vi "MMI_BCM_2A1_Action.vi"(8 "error in":errorcluster caption="错误输入", 9 "Input2":T1, 10 "Input1":T2, 11 "BCM":T3 {"语音命令天窗开关" items=["默认", "停止"]; "天窗开度" scale=0.0..100.0; "右后侧车窗开度" scale=0.0..100.0; "左后侧车窗开度" scale=0.0..100.0; "副驾驶侧车窗开度" scale=0.0..100.0; "伴我回家时间" items=["无", "30s", "60s", "90s"]; "门解锁设置应答" items=["无应答", "应答驾驶门解锁", "应答所有门解锁"]; "天窗翘起控制" items=["无", "倾斜翘起", "倾斜关闭"]; "车窗防夹报警" items=["无", "禁止", "启用"]; "日间行车灯" items=["无", "禁止", "启用"]; "智能弯道灯" items=["无", "禁止", "启用"]; "后视镜自动折叠" items=["无", "禁止", "启用"]; "下雨关窗模式" items=["无", "关", "开"]; "设防提示类型" items=["无", "亮灯并鸣笛", "亮灯", "鸣笛"]; "驾驶侧车窗开度" scale=0.0..100.0}) -> (0 "error out":errorcluster caption="错误输出")   [LabVIEW 2013]
uses:
  MMI_BCM_2A1.ctl
  SendCmdStr/Input1.ctl
  SendCmdStr/Input2.ctl
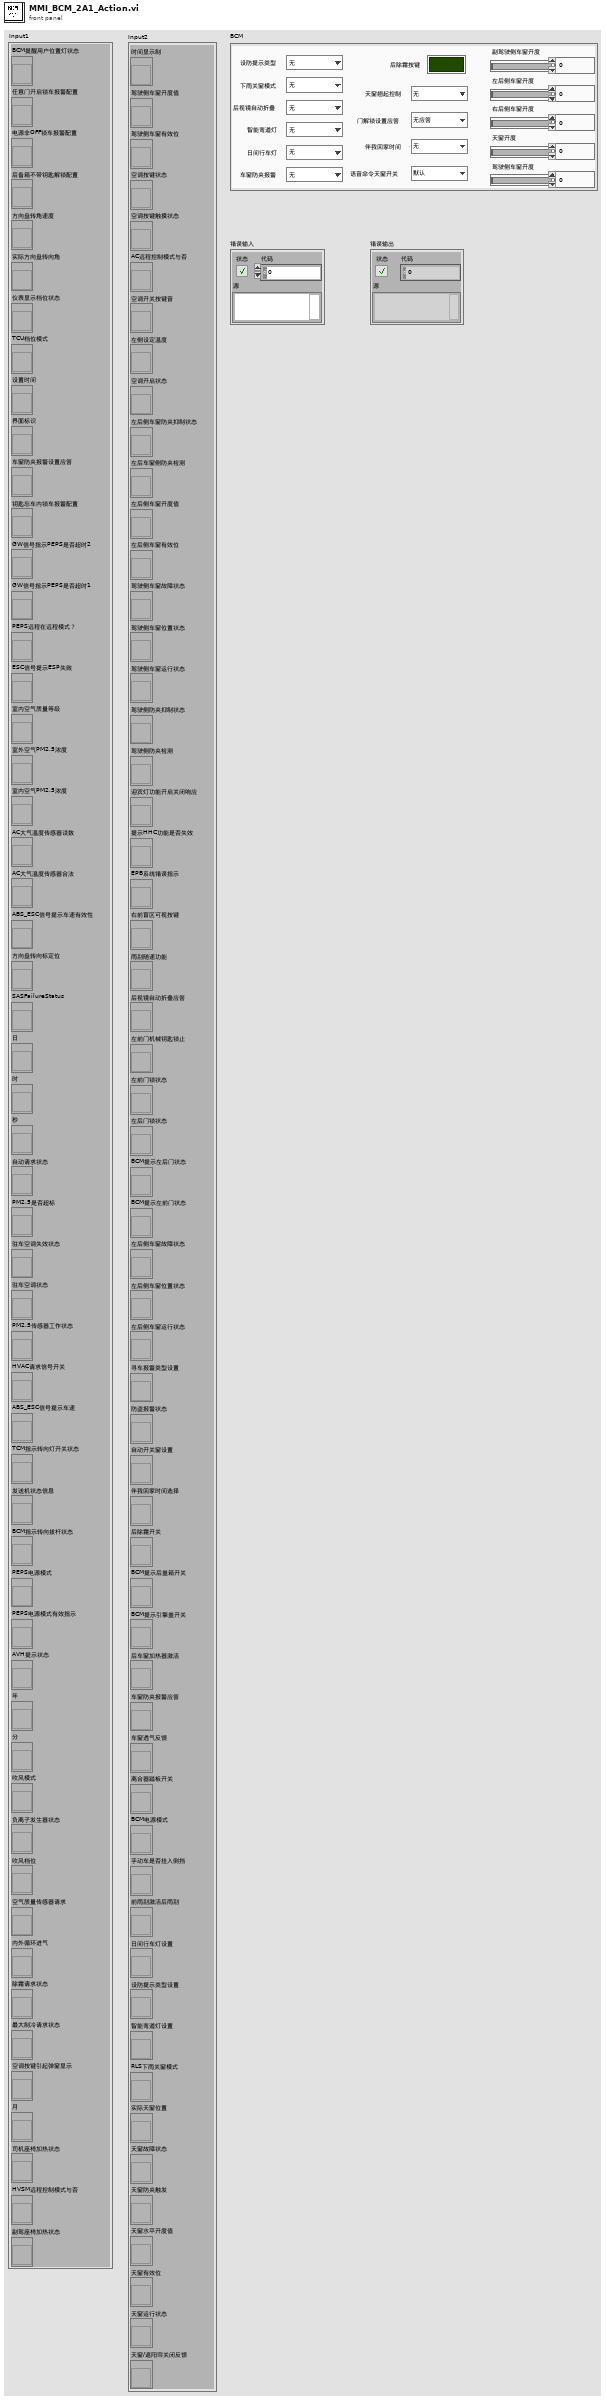
[diagram p1: front panel]
types:
  T1 = typedef "Input2.ctl" = cluster{"时间显示制":refnum<vi>, "驾驶侧车窗开度值":refnum<vi>, "驾驶侧车窗有效位":refnum<vi>, "空调按键状态":refnum<vi>, "空调按键触摸状态":refnum<vi>, "AC远程控制模式与否":refnum<vi>, "空调开关按键音":refnum<vi>, "左侧设定温度":refnum<vi>, "空调开启状态":refnum<vi>, "左后侧车窗防夹抑制状态":refnum<vi>, "左后车窗侧防夹检测":refnum<vi>, "左后侧车窗开度值":refnum<vi>, "左后侧车窗有效位":refnum<vi>, "驾驶侧车窗故障状态":refnum<vi>, "驾驶侧车窗位置状态":refnum<vi>, "驾驶侧车窗运行状态":refnum<vi>, "驾驶侧防夹抑制状态":refnum<vi>, "驾驶侧防夹检测":refnum<vi>, "迎宾灯功能开启关闭响应":refnum<vi>, "提示HHC功能是否失效":refnum<vi>, "EPB系统错误指示":refnum<vi>, "右前盲区可视按键":refnum<vi>, "雨刮随速功能":refnum<vi>, "后视镜自动折叠应答":refnum<vi>, "左前门机械钥匙锁止":refnum<vi>, "左前门锁状态":refnum<vi>, "左后门锁状态":refnum<vi>, "BCM提示左后门状态":refnum<vi>, "BCM提示左前门状态":refnum<vi>, "左后侧车窗故障状态":refnum<vi>, "左后侧车窗位置状态":refnum<vi>, "左后侧车窗运行状态":refnum<vi>, "寻车报警类型设置":refnum<vi>, "防盗报警状态":refnum<vi>, "自动开关窗设置":refnum<vi>, "伴我回家时间选择":refnum<vi>, "后除霜开关":refnum<vi>, "BCM提示后盖箱开关":refnum<vi>, "BCM提示引擎盖开关":refnum<vi>, "后车窗加热器激活":refnum<vi>, "车窗防夹报警应答":refnum<vi>, "车窗透气反馈":refnum<vi>, "离合器踏板开关":refnum<vi>, "BCM电源模式":refnum<vi>, "手动车是否挂入倒挡":refnum<vi>, "前雨刮激活后雨刮":refnum<vi>, "日间行车灯设置":refnum<vi>, "设防提示类型设置":refnum<vi>, "智能弯道灯设置":refnum<vi>, "RLS下雨关窗模式":refnum<vi>, "实际天窗位置":refnum<vi>, "天窗故障状态":refnum<vi>, "天窗防夹触发":refnum<vi>, "天窗水平开度值":refnum<vi>, "天窗有效位":refnum<vi>, "天窗运行状态":refnum<vi>, "天窗/遮阳帘关闭反馈":refnum<vi>}
  T2 = typedef "Input1.ctl" = cluster{"BCM提醒用户位置灯状态":refnum<vi>, "任意门开启锁车报警配置":refnum<vi>, "电源非OFF锁车报警配置":refnum<vi>, "后备箱不带钥匙解锁配置":refnum<vi>, "方向盘转角速度":refnum<vi>, "实际方向盘转向角":refnum<vi>, "仪表显示档位状态":refnum<vi>, "TCU档位模式":refnum<vi>, "设置时间":refnum<vi>, "界面标识":refnum<vi>, "车窗防夹报警设置应答":refnum<vi>, "钥匙忘车内锁车报警配置":refnum<vi>, "GW信号指示PEPS是否超时2":refnum<vi>, "GW信号指示PEPS是否超时1":refnum<vi>, "PEPS远程在远程模式？":refnum<vi>, "ESC信号提示ESP失败":refnum<vi>, "室内空气质量等级":refnum<vi>, "室外空气PM2.5浓度":refnum<vi>, "室内空气PM2.5浓度":refnum<vi>, "AC大气温度传感器读数":refnum<vi>, "AC大气温度传感器合法":refnum<vi>, "ABS_ESC信号提示车速有效性":refnum<vi>, "方向盘转向标定位":refnum<vi>, "SASFailureStatus":refnum<vi>, "日":refnum<vi>, "时":refnum<vi>, "秒":refnum<vi>, "自动请求状态":refnum<vi>, "PM2.5是否超标":refnum<vi>, "驻车空调失效状态":refnum<vi>, "驻车空调状态":refnum<vi>, "PM2.5传感器工作状态":refnum<vi>, "HVAC请求信号开关":refnum<vi>, "ABS_ESC信号提示车速":refnum<vi>, "TCM指示转向灯开关状态":refnum<vi>, "发送机状态信息":refnum<vi>, "BCM指示转向拔杆状态":refnum<vi>, "PEPS电源模式":refnum<vi>, "PEPS电源模式有效指示":refnum<vi>, "AVH提示状态":refnum<vi>, "年":refnum<vi>, "分":refnum<vi>, "吹风模式":refnum<vi>, "负离子发生器状态":refnum<vi>, "吹风档位":refnum<vi>, "空气质量传感器请求":refnum<vi>, "内外循环进气":refnum<vi>, "除霜请求状态":refnum<vi>, "最大制冷请求状态":refnum<vi>, "空调按键引起弹窗显示":refnum<vi>, "月":refnum<vi>, "司机座椅加热状态":refnum<vi>, "HVSM远程控制模式与否":refnum<vi>, "副驾座椅加热状态":refnum<vi>}
  T3 = typedef "MMI_BCM_2A1.ctl" = cluster{"设防提示类型":u16, "下雨关窗模式":u16, "后视镜自动折叠":u16, "智能弯道灯":u16, "日间行车灯":u16, "车窗防夹报警":u16, "天窗翘起控制":u16, "门解锁设置应答":u16, "伴我回家时间":u16, "驾驶侧车窗开度":u8, "后除霜按键":bool, "副驾驶侧车窗开度":u8, "左后侧车窗开度":u8, "右后侧车窗开度":u8, "语音命令天窗开关":u16, "天窗开度":u8}
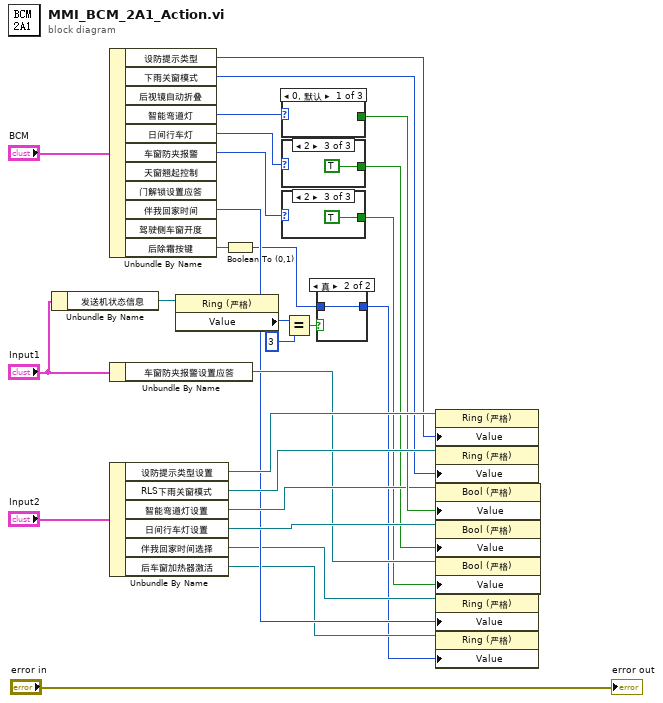
[diagram p0: block diagram]
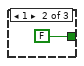
[diagram p4: hidden frame]
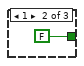
[diagram p6: hidden frame]
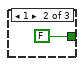
[diagram p7: hidden frame]
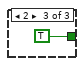
[diagram p8: hidden frame]
diagram:
  n1 = Unbundle By Name("Input1") -> ("发送机状态信息"=w8:refnum<vi>)
  n2 = Unbundle By Name("BCM") -> ("设防提示类型"=w24:u16, "下雨关窗模式"=w22:u16, "智能弯道灯"=w21:u16, "日间行车灯"=w19:u16, "车窗防夹报警"=w15:u16, "伴我回家时间"=w12:u16, "后除霜按键"=w4:bool)  [unwired: 4 out]
  n3 = Unbundle By Name("Input1") -> ("车窗防夹报警设置应答"=w14:refnum<vi>)
  n4 = Unbundle By Name("Input2") -> ("设防提示类型设置"=w25:refnum<vi>, "RLS下雨关窗模式"=w23:refnum<vi>, "智能弯道灯设置"=w18:refnum<vi>, "日间行车灯设置"=w17:refnum<vi>, "伴我回家时间选择"=w11:refnum<vi>, "后车窗加热器激活"=w10:refnum<vi>)
  n5 = property class="Ring (严格)"(reference=w8) -> ("Value"=w7:u16)  [unwired: 1 in, 2 out]
  n6 = Boolean To (0,1)(Boolean=w4) -> (0, 1=w3:i16)
  n7 = case shown="0, 默认" w21 {
    tunnel: [_ FALSE TRUE] -> w20
    frame 0, Default {
    }
    frame 1 {
    }
    frame 2 {
    }
  }
  n8 = case shown="2" w19 {
    tunnel: [_ FALSE TRUE] -> w16
    frame 0, Default {
    }
    frame 1 {
    }
    frame 2 {
    }
  }
  n9 = case shown="2" w15 {
    tunnel: [_ FALSE TRUE] -> w13
    frame 0, Default {
    }
    frame 1 {
    }
    frame 2 {
    }
  }
  n10 = Equal?(x=w7, y=u16 3) -> (x = y?=w5:bool)
  n11 = case shown="真" w5 {
    tunnel: w3 -> [_ w34]
    tunnel: [_ w34] -> w2
    frame False {
    }
    frame True {
    }
  }
  n12 = property class="Ring (严格)"(reference=w25, "Value"=w24) -> ()  [unwired: 1 in, 2 out]
  n13 = property class="Ring (严格)"(reference=w23, "Value"=w22) -> ()  [unwired: 1 in, 2 out]
  n14 = property class="Bool (严格)"(reference=w18, "Value"=w20) -> ()  [unwired: 1 in, 2 out]
  n15 = property class="Bool (严格)"(reference=w17, "Value"=w16) -> ()  [unwired: 1 in, 2 out]
  n16 = property class="Bool (严格)"(reference=w14, "Value"=w13) -> ()  [unwired: 1 in, 2 out]
  n17 = property class="Ring (严格)"(reference=w11, "Value"=w12) -> ()  [unwired: 1 in, 2 out]
  n18 = property class="Ring (严格)"(reference=w10, "Value"=w2) -> ()  [unwired: 1 in, 2 out]
  "error out" <- "error in"
